vi "Insert Value (Single).vi"(7 "key":string, 8 "error in (no error)":errorcluster, 10 "JSON Value in":refnum<class "JSON Value.lvclass">, 11 "JSON Value in":refnum<class "JSON Value.lvclass">) -> (0 "error out":errorcluster, 1 "replaced":bool, 3 "JSON Value out":refnum<class "JSON Value.lvclass">)   [LabVIEW 2016, in "JSON Value.lvclass"]
uses:
  JSON Value.lvclass
  JSON Value.lvclass/JSON Value.ctl
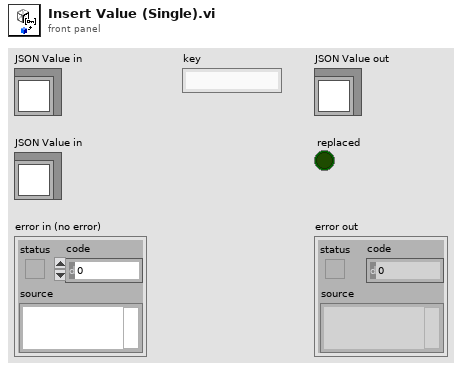
[diagram p1: front panel]
types:
  T1 = typedef "JSON Value.lvclass/JSON Types.ctl" = enum16{"String", "Numeric", "Boolean", "NULL", "Object", "Array"}
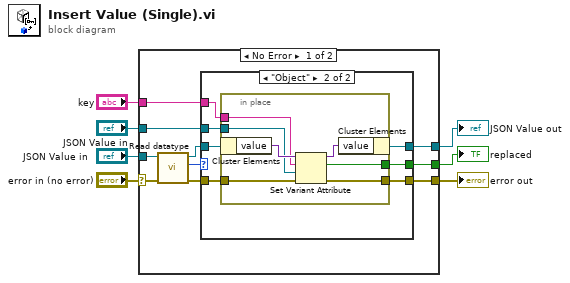
[diagram p0: block diagram]
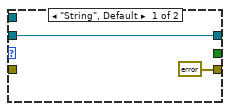
[diagram p2: hidden frame]
diagram:
  n1 = case shown="No Error" "error in (no error)" {
    selector: "error in (no error)" -> [w10 w35]
    tunnel: [w14 w35] -> w2
    tunnel: [w17 w34] -> w4
    tunnel: "JSON Value in" -> [w12 w34]
    tunnel: "key" -> [w16 _]
    tunnel: "JSON Value in" -> [w15 _]
    tunnel: [w13 _] -> w3
    frame No Error {
      n2 = call "Read datatype.vi"("error in (no error)"=w10, "JSON Datatype in"=w12) -> ("error out"=w9:errorcluster, "datatype"=w8:T1, "JSON Datatype out"=w11:refnum<class "JSON Value.lvclass">)  [unwired: 7 in]
      n3 = case shown="\"Object\"" w8 {
        tunnel: [w19 w26] -> w17
        tunnel: w16 -> [_ w25]
        tunnel: w15 -> [_ w24]
        tunnel: [errorcluster {"status"=TRUE, "code"=-1000, "source"="Attempted insert on non-object"} ("error out") w23] -> w14
        tunnel: [_ w22] -> w13
        tunnel: w11 -> [w19 w21]
        tunnel: w9 -> [_ w20]
        frame "String", Default {
        }
        frame "Object" {
          n4 = in-place {
            in-place-border: w25 -> [w32]
            in-place-border: w24 -> [w28]
            in-place-border: w20 -> [w29]
            in-place-border: [w30] -> w23
            in-place-border: [w27] -> w22
            n5 = in-place-cluster #1(w21) -> ("value"=w33:variant)
            n6 = Set Variant Attribute(Variant=w33, name=w32, value=w28, error in=w29) -> (Variant out=w31:variant, replaced=w27:bool, error out=w30:errorcluster)
            n7 = in-place-cluster #1("value"=w31) -> (w26:refnum<class "JSON Value.lvclass">)
          }
        }
      }
    }
    frame Error {
    }
  }
  "error out" <- w2
  "JSON Value out" <- w4
  "replaced" <- w3
